vi "CountAtIndexNow_subvi.vi"(9 "Index Now":i32, 10 "RoundedArray":dbl[](array[numeric]), 11 "hist box in":dbl[](array[numeric])) -> (1 "hist box out":dbl[](array[numeric]), 2 "Count Now":i16)   [LabVIEW 2019]
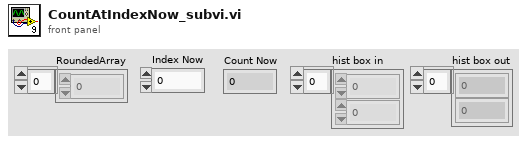
[diagram p1: front panel]
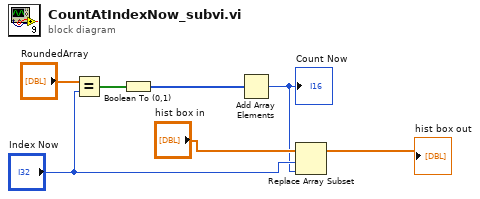
[diagram p0: block diagram]
diagram:
  n1 = Equal?(x="RoundedArray", y="Index Now") -> (x = y?=w5:bool[])
  n2 = Boolean To (0,1)(Boolean=w5) -> (0, 1=w7:i16[])
  n3 = Add Array Elements(numeric array=w7) -> (sum=w2:i16)
  "Count Now" <- w2
  n4 = Replace Array Subset "Replace Array Subset"(array="hist box in", new element=w2, index="Index Now") -> (→"hist box out":dbl[])
